vi "Global Fine procedure.vi"() -> ()   [LabVIEW 2019]
panel:
  out "Fine procedure?":bool
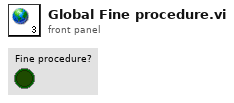
[diagram p1: front panel]
diagram:
